vi "Rodrigues.vi"   [LabVIEW 2020, in "ar.lvlib"]
uses:
  ar.lvlib
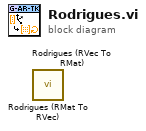
[diagram p0: block diagram]
diagram:
  n1 = call "Rodrigues (RMat To RVec).vi"() -> ()  [unwired: 10 in, 2 out]
  n2 = call "Rodrigues (RVec To RMat).vi"() -> ()  [unwired: 10 in, 2 out]
